vi "Test_freq_generator.vi"() -> ()   [LabVIEW 2013]
panel:
  out "Waveform Graph":dbl[][](graph)
  out "hi(x) 4":fxp<+/-,16,0> format="%016b"
  out "hi(x) 3":fxp<+/-,16,0> format="%016b"
  out "hi(x) 2":u16 format="%016b"
  out "Array 2":fxp<+/-,16,0>[](array[numeric]) format="%.16g"
  out "hi(x)":u16 format="%016b"
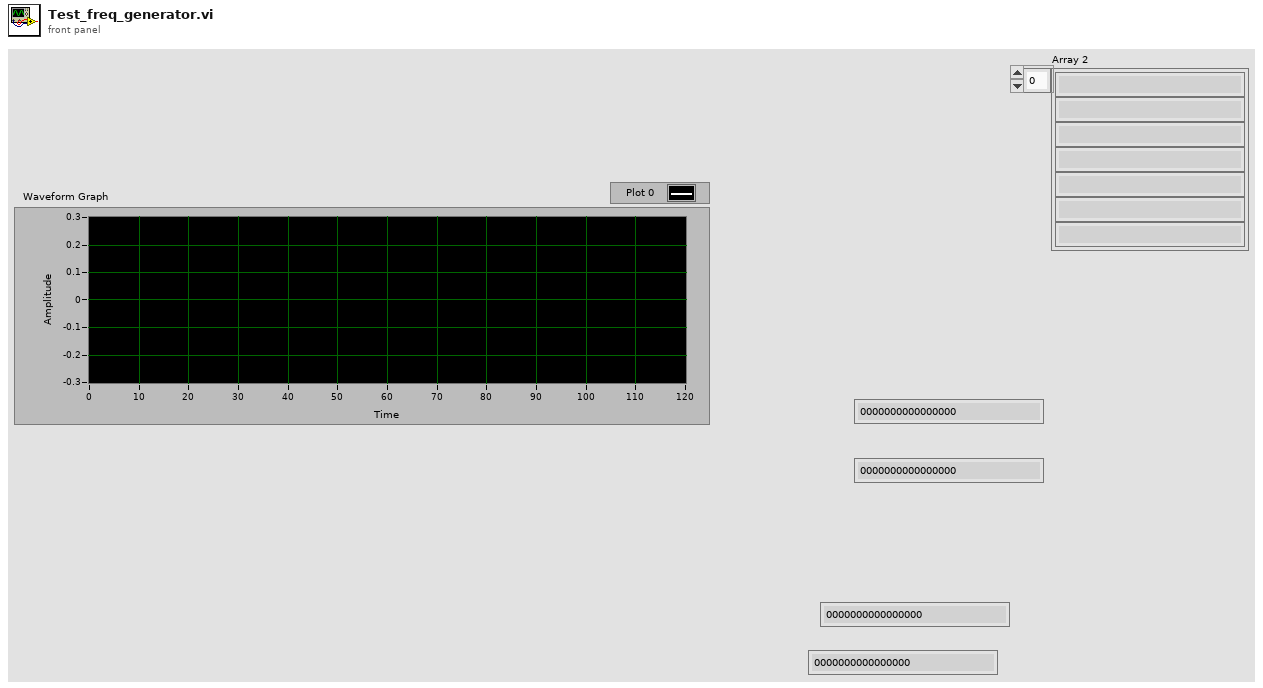
[diagram p1: front panel]
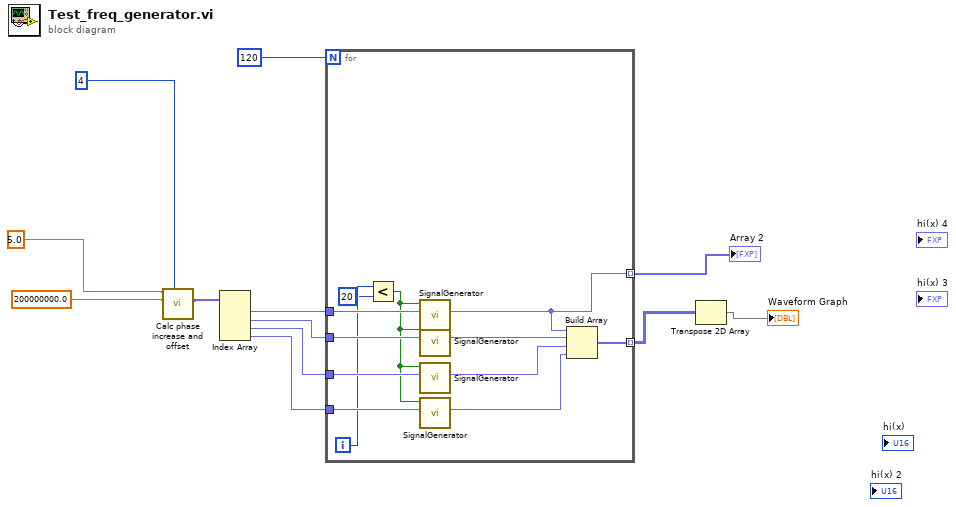
[diagram p0: block diagram]
diagram:
  n1 = call "Calc phase increase and offset.vi"("# of DDS"=4, "fclk (800MHz)"=200000000.0, "f_generated (MHz)"=5.0) -> ("Phase out"=w1:fxp<+,64,64>[])  [unwired: 6 in, 2 out]
  n2 = Index Array(array=w1) -> (element #1=w10:fxp<+,64,64>, element #2=w7:fxp<+,64,64>, element #3=w6:fxp<+,64,64>, element #4=w5:fxp<+,64,64>)  [unwired: 4 in]
  n3 = for {
    N: 120 -> [_]
    tunnel: w10 -> [w24]
    tunnel: w7 -> [w23]
    tunnel: w6 -> [w22]
    tunnel: w5 -> [w21]
    tunnel: [w20] -> w11 mode=indexing
    tunnel: [w18] -> w9 mode=indexing
    i -> [w15]
    n4 = Less?(x=w15, y=20) -> (x < y?=w13:bool)
    n5 = call "SignalGenerator.vi"("phase"=w24, "Reset"=w13) -> ("Sin"=w18:fxp<+/-,16,0>)  [unwired: 7 in, 2 out]
    n6 = call "SignalGenerator.vi"("phase"=w23, "Reset"=w13) -> ("Sin"=w19:fxp<+/-,16,0>)  [unwired: 7 in, 2 out]
    n7 = call "SignalGenerator.vi"("phase"=w22, "Reset"=w13) -> ("Sin"=w17:fxp<+/-,16,0>)  [unwired: 7 in, 2 out]
    n8 = call "SignalGenerator.vi"("phase"=w21, "Reset"=w13) -> ("Sin"=w16:fxp<+/-,16,0>)  [unwired: 7 in, 2 out]
    n9 = Build Array(w18, w19, w17, w16) -> (w20:fxp<+/-,16,0>[])
  }
  "Array 2" <- w9
  n10 = Transpose 2D Array(2D array=w11) -> (transposed array=→"Waveform Graph":fxp<+/-,16,0>[][])
